vi "Update Class Name.vi"(8 "error in (no error)":errorcluster, 10 "Class Name":string, 11 "ControlClassWizard in":refnum<class "QControl Creation Wizard.lvclass">) -> (0 "error out":errorcluster, 1 "Banner Text":string, 2 "Localized Name":string, 3 "ControlClassWizard out":refnum<class "QControl Creation Wizard.lvclass">, 4 "New Class Folder Path":path, 5 "Final Path":string)   [LabVIEW 2015, in "QControl Creation Wizard.lvclass"]
doc: "<b> </b> <b> </b>\n©2016 Q Software Innovations, LLC (QSI)\nwritten by Quentin Alldredge\nproduced in LabVIEW 2015\n\nsupport@qsoftwareinnovations.com\nwww.qsoftwareinnovations.com\n\nAll rights reserved.\n\nRedistribution and use in source and binary forms, with or without modification, are permitted provided that the following conditions are met:\n\n * Redistributions of source code must retain the above copyright notice, this list of conditions and the following disclaimer.\n * Redistributions in binary form must reproduce the above copyright notice, this list of conditions and the following disclaimer in the documentation and/or other materials provided with the distribution.\n * Neither the name of Q Software Innovations, LLC. nor the names of its contributors may be used to endorse or promote products derived from this software without specific prior written permission.\n\nTHIS SOFTWARE IS PROVIDED BY THE COPYRIGHT HOLDERS AND CONTRIBUTORS \"AS IS\" AND ANY EXPRESS OR IMPLIED WARRANTIES, INCLUDING, BUT NOT LIMITED TO, THE IMPLIED WARRANTIES OF MERCHANTABILITY AND FITNESS FOR A PARTICULAR PURPOSE ARE DISCLAIMED. IN NO EVENT SHALL THE COPYRIGHT OWNER OR CONTRIBUTORS BE LIABLE FOR ANY DIRECT, INDIRECT, INCIDENTAL, SPECIAL, EXEMPLARY, OR CONSEQUENTIAL DAMAGES (INCLUDING, BUT NOT LIMITED TO, PROCUREMENT OF SUBSTITUTE GOODS OR SERVICES; LOSS OF USE, DATA, OR PROFITS; OR BUSINESS INTERRUPTION) HOWEVER CAUSED AND ON ANY THEORY OF LIABILITY, WHETHER IN CONTRACT, STRICT LIABILITY, OR TORT (INCLUDING NEGLIGENCE OR OTHERWISE) ARISING IN ANY WAY OUT OF THE USE OF THIS SOFTWARE, EVEN IF ADVISED OF THE POSSIBILITY OF SUCH DAMAGE."
uses:
  QControl Creation Wizard.lvclass
  QControl Creation Wizard.lvclass/QControl Creation Wizard.ctl
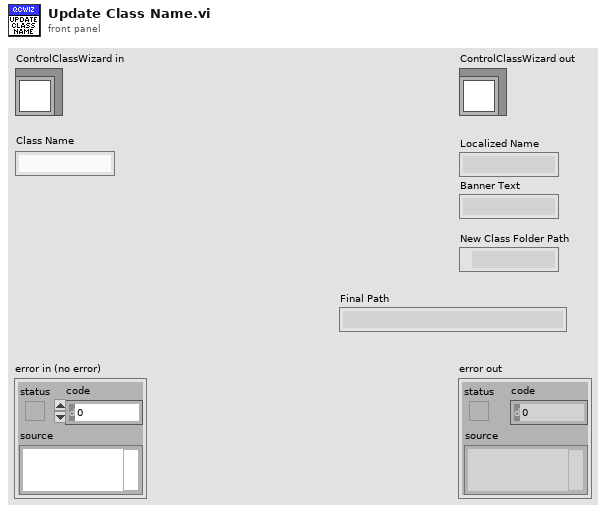
[diagram p1: front panel]
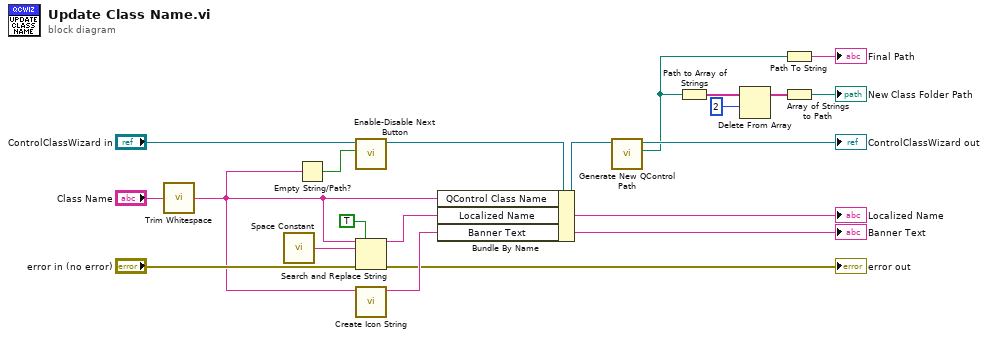
[diagram p0: block diagram]
diagram:
  n1 = call <vilib>:"Trim Whitespace.vi"("string"="Class Name") -> ("trimmed string"=w2:string)  [unwired: 1 in]
  n2 = call <vilib>:"Space Constant.vi"() -> ("String"=w16:string)
  n3 = Empty String/Path?(string/path=w2) -> (empty?=w1:bool)
  n4 = call "Enable-Disable Next Button.vi"("Disable Next Button?"=w1, "QControlWizard in"="ControlClassWizard in") -> ("QControlWizard (dup)"=w8:refnum<class "QControl Creation Wizard.lvclass">)  [unwired: 8 in, 1 out]
  n5 = Search and Replace String(replace all?=TRUE ("replace all? (F)"), input string=w2, search string=w16, error in="error in (no error)") -> (result string=w19:string, error out=→"error out":errorcluster)  [unwired: 4 in, 2 out]
  "Localized Name" <- w19
  n6 = call "Create Icon String.vi"("Simple Class Name"=w2) -> ("Abbriviated Icon Name"=w18:string)  [unwired: 10 in]
  "Banner Text" <- w18
  n7 = Bundle By Name(cluster=w8, "QControl Class Name"=w2, "Localized Name"=w19, "Banner Text"=w18) -> (w5:refnum<class "QControl Creation Wizard.lvclass">)
  n8 = call "Generate New QControl Path.vi"("QControl Wizard in"=w5) -> ("New Class Path"=w3:path, "QControl Wizard out"=→"ControlClassWizard out":refnum<class "QControl Creation Wizard.lvclass">)  [unwired: 8 in, 1 out]
  n9 = Path to Array of Strings(0:w3) -> (2:w14:string[])  [unwired: 1 out]
  n10 = Delete From Array(array=w14, length=2) -> (array with subset deleted=w12:string[])  [unwired: 1 in, 1 out]
  n11 = Path To String(path=w3) -> (string=→"Final Path":string)
  n12 = Array of Strings to Path(0:w12) -> (2:→"New Class Folder Path":path)  [unwired: 1 in]
